vi "Untitled 17.vi"() -> ()   [LabVIEW 2012]
uses:
  <vilib>/Utility/NIReport.llb/NI_report.lvclass
  <vilib>/addons/database/Auxilliary.llb/DB Tools Cursor Type.ctl
  <vilib>/addons/_office/_exclsub.llb/font.ctl
  <vilib>/addons/_office/excel.llb/Excel Get Data (str).vi
  <vilib>/addons/database/Connection.llb/DB Tools Open Connec (Path).vi
  <vilib>/addons/database/Connection.llb/Conn Execute.vi
  <vilib>/addons/database/Recordset.llb/Rec Fetch Recordset Data (R).vi
  <vilib>/addons/database/Recordset.llb/Rec Destroy - Connection.vi
  <vilib>/Utility/NIReport.llb/Excel/NI_Excel.lvclass
  <vilib>/addons/_office/NI_ReportGenerationToolkit.lvlib
  <vilib>/addons/database/NI_Database_API.lvlib
panel:
  out "recordset data":variant[][](array[variant])
  out "error out 5":errorcluster
  out "error out 3":errorcluster
  out "error out 2":errorcluster
  out "source":string
  out "error out":errorcluster
  out "concatenated string 2":string
  in  "start (0, 0) 4":cluster{"start row":i32, "start column":i32}
  out "concatenated string":string
  in  "start (0, 0) 3":cluster{"start row":i32, "start column":i32}
  out "Numeric":i32
  out "ExcelRow":i32
  in  "start (0, 0)":cluster{"start row":i32, "start column":i32}
  out "x+y":i32
  out "data":string
  in  "start (0, 0) 2":cluster{"start row":i32, "start column":i32}
  out "row":i32
  out "array":string[][](array[string])
  out "error out 4":errorcluster
  out "spreadsheet string":string
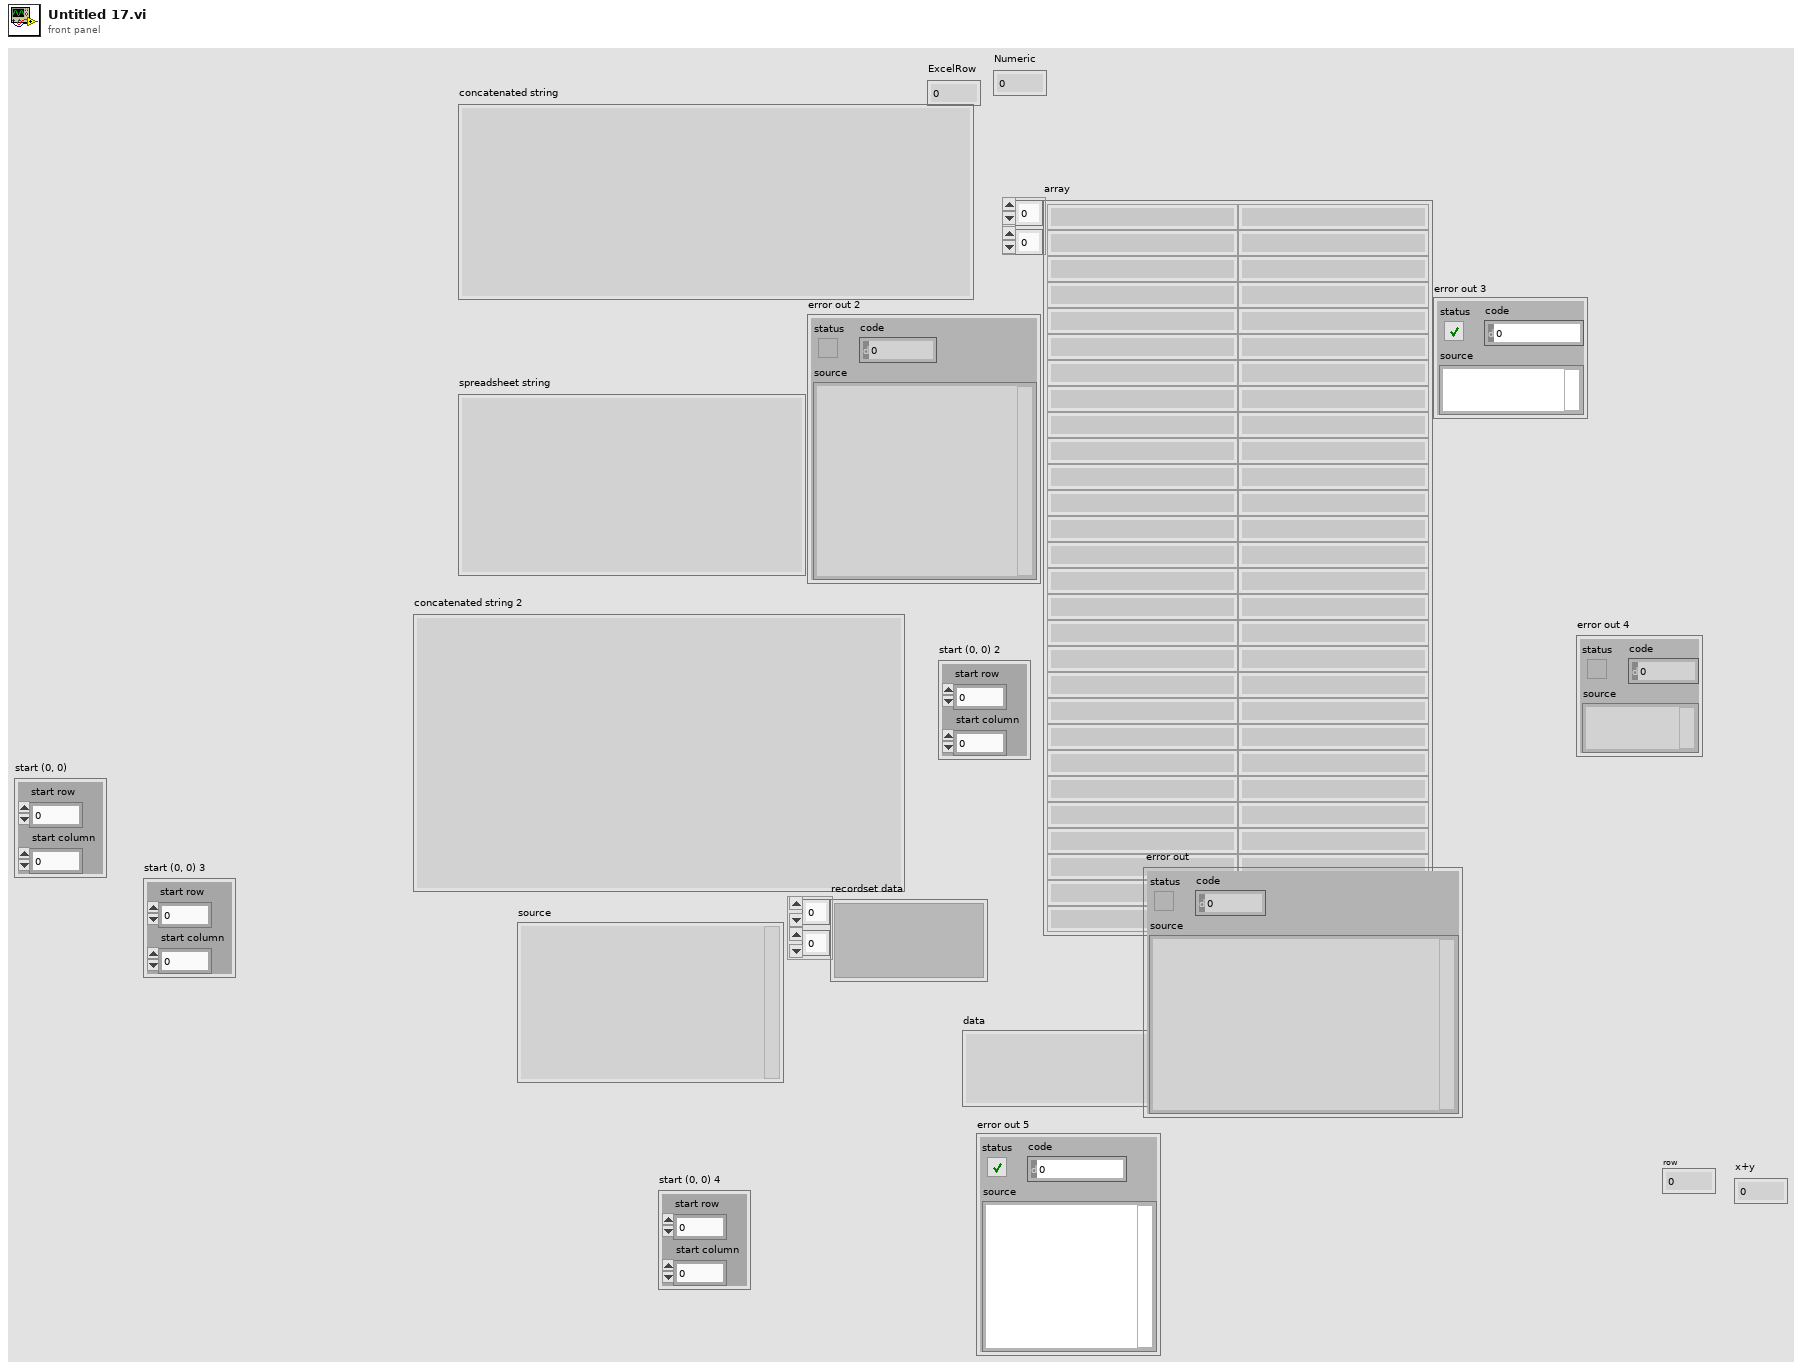
[diagram p1: front panel]
types:
  T1 = enum16{"Standard Report", "HTML", "Word", "Excel"}
  T2 = typedef "NI_ReportGenerationToolkit.lvlib/font.ctl" = cluster{"font name":string, "font size":dbl, "bold":u16, "italic":u16, "underline":u16, "strike through":u16, "font color":u32}
  T3 = cluster{"on/off":bool, "weight":i32, "color":u32}
  T4 = typedef "NI_Database_API.lvlib/DB Tools Cursor Type.ctl" = enum16{"forward-only", "keyset", "dynamic", "static"}
  T5 = typedef "NI_Database_API.lvlib/Conn ObjectReference.ctl" = refnum<k1>
  T6 = typedef "NI_Database_API.lvlib/Rec ObjectReference.ctl" = refnum<k1>
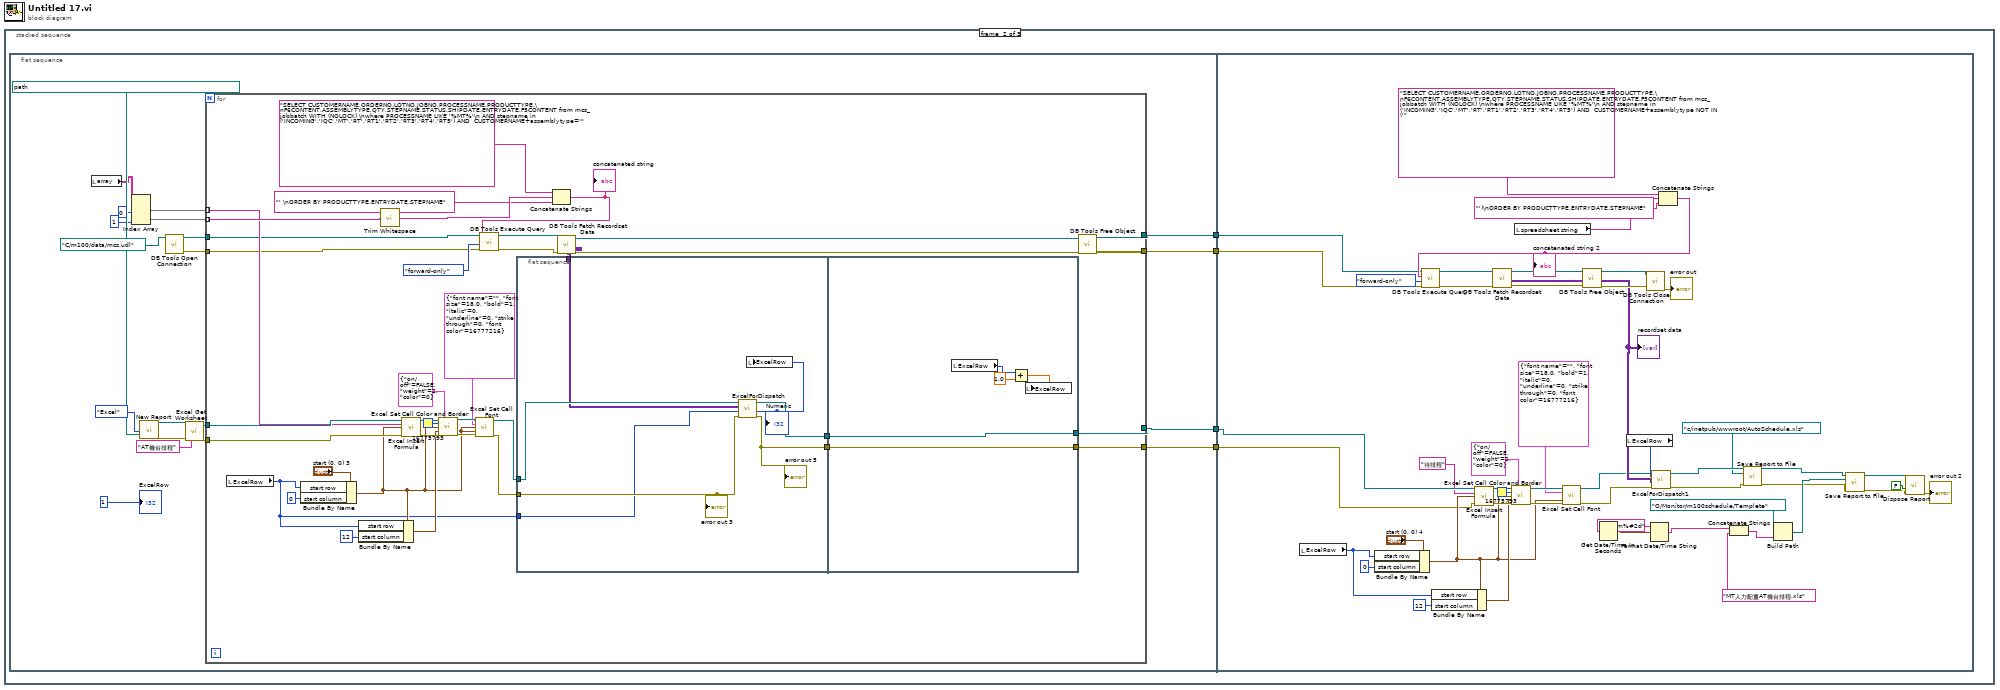
[diagram p0: block diagram]
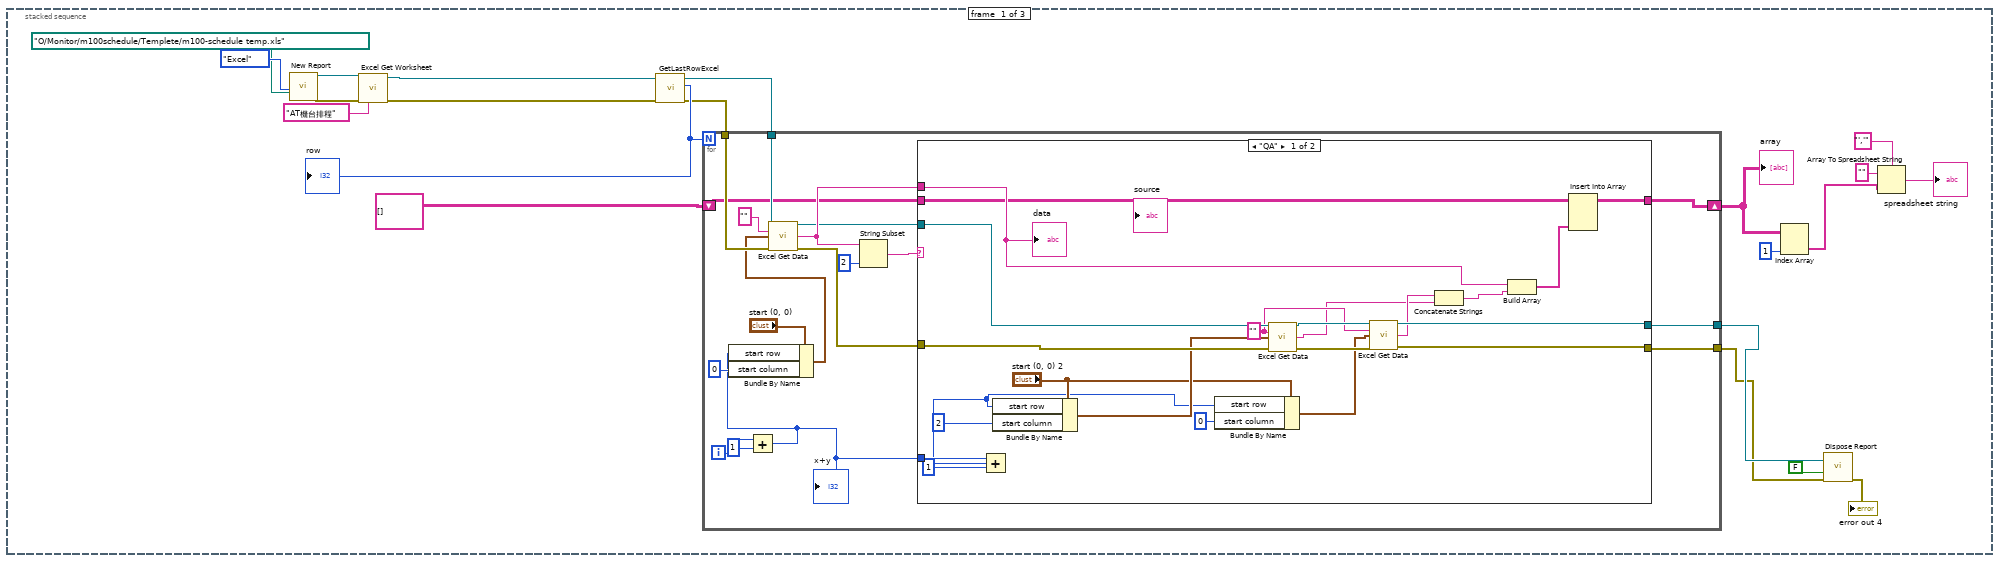
[diagram p2: hidden frame]
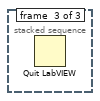
[diagram p4: hidden frame]
diagram:
  n1 = stacked-sequence {
    frame #0 {
      n2 = call <vilib>:"New Report.vi"("report type"=T1."Excel" ("Report Type"), "template (empty)"=path "O:/Monitor/m100schedule/Templete/m100-schedule temp.xls") -> ("report out"=w20:refnum<class "NI_report.lvclass">, "error out"=w19:errorcluster)  [unwired: 12 in]
      n3 = call <vilib>:"Excel Get Worksheet.vi"("report in"=w20, "error in (no error)"=w19, "name (\"\")"="AT機台排程" ("name (\"\")")) -> ("report out"=w18:refnum<class "NI_report.lvclass">, "error out"=w17:errorcluster)  [unwired: 11 in]
      n4 = call "GetLastRowExcel.vi"("error in (no error)"=w17, "report in"=w18) -> ("error out"=w13:errorcluster, "row"=w16:i32, "report out"=w12:refnum<class "NI_report.lvclass">)  [unwired: 7 in]
      "row" <- w16
      n5 = for {
        N: w16 -> [_]
        tunnel: w12 -> [w39]
        tunnel: w13 -> [w38]
        shift-right: [w27] -> w3
        shift-left: string[][] [] ("array") -> [w28]
        tunnel: [w23] -> w8
        tunnel: [w22] -> w7
        i -> [w34]
        n6 = Add(x=w34, y=1) -> (x+y=w24:i32)
        "x+y" <- w24
        n7 = Bundle By Name(cluster="start (0, 0)", "start row"=w24, "start column"=0) -> (w35:cluster{"start row":i32, "start column":i32})
        n8 = call-poly <vilib>:"Excel Get Data.vi"("report in"=w39, "data type"="", "start (0, 0)"=w35, "error in (no error)"=w38) -> ("report out"=w26:refnum<class "NI_report.lvclass">, "data"=w30:string, "error out"=w25:errorcluster)  [unwired: 9 in]
        n9 = String Subset(string=w30, length (rest)=2 ("length (rest)")) -> (substring=w31:string)  [unwired: 1 in]
        n10 = case shown="\"QA\"" w31 {
          tunnel: w30 -> [w61 _]
          tunnel: w28 -> [w58 w64]
          tunnel: [w59 w64] -> w27
          tunnel: w26 -> [w57 w63]
          tunnel: w25 -> [w56 w62]
          tunnel: w24 -> [w53 _]
          tunnel: [w49 w63] -> w23
          tunnel: [w48 w62] -> w22
          frame "QA" {
            w47 = "" ("data type")
            n11 = Add(x=w53, y=1) -> (x+y=w45:i32)
            n12 = Bundle By Name(cluster="start (0, 0) 2", "start row"=w45, "start column"=2) -> (w55:cluster{"start row":i32, "start column":i32})
            n13 = Bundle By Name(cluster="start (0, 0) 2", "start row"=w45, "start column"=0) -> (w43:cluster{"start row":i32, "start column":i32})
            n14 = call-poly <vilib>:"Excel Get Data.vi"("report in"=w57, "data type"=w47, "start (0, 0)"=w55, "error in (no error)"=w56) -> ("report out"=w51:refnum<class "NI_report.lvclass">, "data"=w41:string, "error out"=w50:errorcluster)  [unwired: 9 in]
            n15 = call-poly <vilib>:"Excel Get Data.vi"("report in"=w51, "data type"=w47, "start (0, 0)"=w43, "error in (no error)"=w50) -> ("report out"=w49:refnum<class "NI_report.lvclass">, "data"=w42:string, "error out"=w48:errorcluster)  [unwired: 9 in]
            n16 = Concatenate Strings(w42, w41) -> (w40:string)
            n17 = Build Array(w61, w40) -> (w60:string[])
            n18 = Insert Into Array(array=w58, new element=w60) -> (w59:string[][])  [unwired: 2 in]
            "data" <- w61
          }
          frame Default {
          }
        }
      }
      "array" <- w3
      n19 = Index Array(array=w3, index (col)=1 ("disabled index (col)")) -> (element=w1:string[])  [unwired: 1 in]
      n20 = call-dynamic "Dispose Report.vi"("report in"=w8, "save changes? (F)"=FALSE, "error in (no error)"=w7) -> ("error out"=→"error out 4":errorcluster)  [unwired: 12 in]
      n21 = Array To Spreadsheet String(delimiter (Tab)="','", array=w1, 3:"" ("format string")) -> (spreadsheet string=→"spreadsheet string":string)
    }
    frame #1 {
      n22 = flat-sequence {
        tunnel: [w72] -> w68
        tunnel: [w71] -> w67
        tunnel: [w70] -> w66
        tunnel: [w69] -> w65
        tunnel: w68 -> [w174]
        tunnel: w67 -> [w173]
        tunnel: w66 -> [w146]
        tunnel: w65 -> [w138]
        frame #0 {
          n23 = local read "array"() -> (w83:string[][])
          n24 = Index Array(array=w83, index (col) #1=0 ("disabled index (col)"), index (col) #2=1 ("index (col)")) -> (element #1=w82:string[], element #2=w79:string[])  [unwired: 2 in]
          n25 = call <vilib>:"New Report.vi"("report type"=T1."Excel" ("Report Type"), "template (empty)"=path "O:/Monitor/m100schedule/Templete/MT人力配置AT機台排程.xls" ("template (empty) 2")) -> ("report out"=w87:refnum<class "NI_report.lvclass">, "error out"=w86:errorcluster)  [unwired: 12 in]
          n26 = call-poly <vilib>:"DB Tools Open Connection.vi"("connection information"=path "C:/m100/data/mcs.udl") -> ("error out"=w73:errorcluster, "connection reference"=w74:T5)  [unwired: 7 in]
          n27 = call <vilib>:"Excel Get Worksheet.vi"("report in"=w87, "error in (no error)"=w86, "name (\"\")"="AT機台排程" ("name (\"\")")) -> ("report out"=w78:refnum<class "NI_report.lvclass">, "error out"=w77:errorcluster)  [unwired: 11 in]
          n28 = for {
            tunnel: w82 -> [w113] mode=indexing
            tunnel: w79 -> [w118] mode=indexing
            tunnel: w78 -> [w115]
            tunnel: w77 -> [w114]
            tunnel: [w98] -> w70
            tunnel: w74 -> [w97]
            tunnel: w73 -> [w96]
            tunnel: [w95] -> w72
            tunnel: [w94] -> w71
            tunnel: [w90] -> w69
            n29 = local read "ExcelRow"() -> (w92:i32)
            n30 = Bundle By Name(cluster="start (0, 0) 3", "start row"=w92, "start column"=0) -> (w100:cluster{"start row":i32, "start column":i32})
            n31 = Bundle By Name(cluster=w100, "start row"=w92, "start column"=12) -> (w105:cluster{"start row":i32, "start column":i32})
            n32 = call <vilib>:"Trim Whitespace.vi"("string"=w118) -> ("trimmed string"=w117:string)  [unwired: 1 in]
            n33 = call <vilib>:"Excel Insert Formula.vi"("report in"=w115, "formula"=w113, "start (0, 0)"=w100, "error in (no error)"=w114) -> ("report out"=w110:refnum<class "NI_report.lvclass">, "error out"=w109:errorcluster)  [unwired: 10 in]
            n34 = call <vilib>:"Excel Set Cell Color and Border.vi"("report in"=w110, "inside border"=T3 {"on/off"=FALSE, "weight"=2, "color"=0}, "background color (w)"=u32 16775793, "start (-1, -1)"=w100, "end (-1, -1)"=w105, "error in (no error)"=w109) -> ("report out"=w104:refnum<class "NI_report.lvclass">, "error out"=w103:errorcluster)  [unwired: 8 in]
            n35 = call <vilib>:"Excel Set Cell Font.vi"("report in"=w104, "font"=T2 {"font name"="", "font size"=18.0, "bold"=1, "italic"=0, "underline"=0, "strike through"=0, "font color"=16777216}, "start (-1, -1)"=w100, "end (-1, -1)"=w100, "error in (no error)"=w103) -> ("report out"=w102:refnum<class "NI_report.lvclass">, "error out"=w101:errorcluster)  [unwired: 9 in]
            n36 = flat-sequence {
              tunnel: w116 -> [w130]
              tunnel: w102 -> [w132]
              tunnel: w101 -> [w131]
              tunnel: [w129] -> w93
              tunnel: w92 -> [w127]
              tunnel: [w126] -> w89
              tunnel: [w134] -> w98
              tunnel: w93 -> [w134]
              tunnel: [w133] -> w90
              tunnel: w89 -> [w133]
              frame #0 {
                n37 = call "ExcelForDispatch.vi"("error out"=w131, "RowNo"=w127, "array"=w130, "report out"=w132) -> ("error out 2"=w126:errorcluster, "Numeric"=w128:i32, "report out 2"=w129:refnum<class "NI_report.lvclass">)  [unwired: 5 in]
                "Numeric" <- w128
                "error out 5" <- w126
                n38 = local write "ExcelRow"(w128) -> ()
                "error out 3" <- w131
              }
              frame #1 {
                n39 = local read "ExcelRow"() -> (w136:i32)
                n40 = Add(x=w136, y=1.0) -> (x+y=w135:dbl)
                n41 = local write "ExcelRow"(w135) -> ()
              }
            }
            n42 = Concatenate Strings("SELECT CUSTOMERNAME,ORDERNO,LOTNO,JOBNO,PROCESSNAME,PRODUCTTYPE,\nF6CONTENT,ASSEMBLYTYPE,QTY,STEPNAME,STATUS,SHIPDATE,ENTRYDATE,F5CONTENT from mcs_jobbatch WITH (NOLOCK) \nwhere PROCESSNAME LIKE '%MT%'\n AND stepname in ('INCOMING','IQC','MT','RT','RT1','RT2','RT3','RT4','RT5') AND  CUSTOMERNAME+assemblytype='" ("SQL query"), w117, "' \nORDER BY PRODUCTTYPE,ENTRYDATE,STEPNAME" ("string")) -> (w120:string)
            "concatenated string" <- w120
            n43 = call-poly <vilib>:"DB Tools Execute Query.vi"("error in (no error)"=w96, "cursor type"=DB_Tools_Cursor_Type."forward-only", "SQL query"=w120, "connection reference"=w97) -> ("error out"=w123:errorcluster, "recordset reference"=w125:T6)  [unwired: 4 in]
            n44 = call-poly <vilib>:"DB Tools Fetch Recordset Data.vi"("error in (no error)"=w123, "recordset reference"=w125) -> ("error out"=w122:errorcluster, "recordset data"=w116:variant[][], "recordset reference out"=w124:T6)  [unwired: 3 in]
            n45 = call-poly <vilib>:"DB Tools Free Object.vi"("error in (no error)"=w122, "recordset reference"=w124) -> ("error out"=w94:errorcluster, "connection reference"=w95:T5)  [unwired: 8 in]
          }
          "ExcelRow" <- 1
        }
        frame #1 {
          n46 = local read "ExcelRow"() -> (w149:i32)
          n47 = Bundle By Name(cluster="start (0, 0) 4", "start row"=w149, "start column"=0) -> (w151:cluster{"start row":i32, "start column":i32})
          n48 = Bundle By Name(cluster=w151, "start row"=w149, "start column"=12) -> (w154:cluster{"start row":i32, "start column":i32})
          n49 = call <vilib>:"Excel Insert Formula.vi"("report in"=w146, "formula"="待排程", "start (0, 0)"=w151, "error in (no error)"=w138) -> ("report out"=w159:refnum<class "NI_report.lvclass">, "error out"=w158:errorcluster)  [unwired: 10 in]
          n50 = call <vilib>:"Excel Set Cell Color and Border.vi"("report in"=w159, "inside border"=T3 {"on/off"=FALSE, "weight"=2, "color"=0}, "background color (w)"=u32 16775793, "start (-1, -1)"=w151, "end (-1, -1)"=w154, "error in (no error)"=w158) -> ("report out"=w153:refnum<class "NI_report.lvclass">, "error out"=w152:errorcluster)  [unwired: 8 in]
          n51 = local read "spreadsheet string"() -> (w179:string)
          n52 = call <vilib>:"Excel Set Cell Font.vi"("report in"=w153, "font"=T2 {"font name"="", "font size"=18.0, "bold"=1, "italic"=0, "underline"=0, "strike through"=0, "font color"=16777216}, "start (-1, -1)"=w151, "end (-1, -1)"=w151, "error in (no error)"=w152) -> ("report out"=w148:refnum<class "NI_report.lvclass">, "error out"=w147:errorcluster)  [unwired: 9 in]
          n53 = Get Date/Time In Seconds() -> (seconds since 1Jan1904=w164:timestamp)
          n54 = local read "ExcelRow"() -> (w175:i32)
          n55 = Format Date/Time String(time format string (%c)="%#2m%#2d", seconds (now)=w164) -> (date/time string=w162:string)  [unwired: 1 in]
          n56 = Concatenate Strings("SELECT CUSTOMERNAME,ORDERNO,LOTNO,JOBNO,PROCESSNAME,PRODUCTTYPE,\nF6CONTENT,ASSEMBLYTYPE,QTY,STEPNAME,STATUS,SHIPDATE,ENTRYDATE,F5CONTENT from mcs_jobbatch WITH (NOLOCK) \nwhere PROCESSNAME LIKE '%MT%'\n AND stepname in ('INCOMING','IQC','MT','RT','RT1','RT2','RT3','RT4','RT5') AND  CUSTOMERNAME+assemblytype NOT IN ('" ("SQL query"), w179, "')\nORDER BY PRODUCTTYPE,ENTRYDATE,STEPNAME" ("string")) -> (w177:string)
          "concatenated string 2" <- w177
          n57 = call-poly <vilib>:"DB Tools Execute Query.vi"("error in (no error)"=w173, "cursor type"=DB_Tools_Cursor_Type."forward-only", "SQL query"=w177, "connection reference"=w174) -> ("error out"=w185:errorcluster, "recordset reference"=w187:T6)  [unwired: 4 in]
          n58 = call-poly <vilib>:"DB Tools Fetch Recordset Data.vi"("error in (no error)"=w185, "recordset reference"=w187) -> ("error out"=w184:errorcluster, "recordset data"=w176:variant[][], "recordset reference out"=w186:T6)  [unwired: 3 in]
          "recordset data" <- w176
          n59 = call-poly <vilib>:"DB Tools Free Object.vi"("error in (no error)"=w184, "recordset reference"=w186) -> ("error out"=w183:errorcluster, "connection reference"=w182:T5)  [unwired: 8 in]
          n60 = call <vilib>:"DB Tools Close Connection.vi"("error in (no error)"=w183, "connection reference"=w182) -> ("error out"=→"error out":errorcluster)  [unwired: 5 in]
          n61 = call "ExcelForDispatch1.vi"("error out"=w147, "RowNo"=w175, "array"=w176, "report out"=w148) -> ("error out 2"=w143:errorcluster, "report out 2"=w144:refnum<class "NI_report.lvclass">)  [unwired: 6 in]
          n62 = Concatenate Strings(w162, "MT人力配置AT機台排程.xls" ("string")) -> (w166:string)
          n63 = call-dynamic "Save Report to File.vi"("report in"=w144, "report file path"=path "c:/inetpub/wwwroot/AutoSchedule.xls", "error in (no error)"=w143) -> ("report out"=w142:refnum<class "NI_report.lvclass">, "error out"=w141:errorcluster)  [unwired: 11 in]
          n64 = Build Path(base path=path "O:/Monitor/m100schedule/Templete", name or relative path=w166) -> (appended path=w167:path)
          n65 = call-dynamic "Save Report to File.vi"("report in"=w142, "report file path"=w167, "error in (no error)"=w141) -> ("report out"=w169:refnum<class "NI_report.lvclass">, "error out"=w168:errorcluster)  [unwired: 11 in]
          n66 = call-dynamic "Dispose Report.vi"("report in"=w169, "save changes? (F)"=FALSE, "error in (no error)"=w168) -> ("error out"=→"error out 2":errorcluster)  [unwired: 12 in]
        }
      }
    }
    frame #2 {
      n67 = Quit LabVIEW() -> ()  [unwired: 1 in]
    }
  }
